vi "load Defects Script.vi"(8 "error in (no error)":errorcluster) -> (0 "error out":errorcluster)   [LabVIEW 2019, in "defectsWrapper.lvlib"]
doc: "void loadDefectsScript(void)"
uses:
  defectsWrapper.lvlib
  defectsWrapper.dll
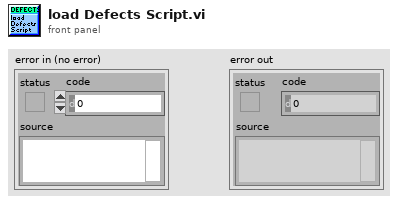
[diagram p1: front panel]
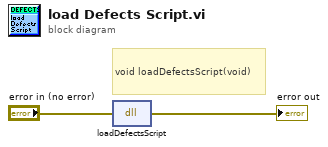
[diagram p0: block diagram]
diagram:
  # "void loadDefectsScript(void)"
  n1 = dll-call lib="C:/Users/user/Desktop/defectsWrapper2/defectsWrapper.*" fn="loadDefectsScript"(error in="error in (no error)") -> (error out=→"error out":errorcluster)  [unwired: 3 in, 1 out]
